vi "Ethernet Packet Generator for Testing.vi"() -> ()   [LabVIEW 2025]
uses:
  <vilib>/xnet/xnet.llb/XNET Frame Type Ethernet.ctl
  <vilib>/xnet/xnet.llb/XNET Create Session (Frame Output Stream).vi
  <vilib>/xnet/xnet.llb/XNET Write (Frame Ethernet).vi
  Automotive Ethernet Bus Monitor/Automotive Ethernet Bus Monitor.lvclass
panel:
  out "error out":errorcluster
  in  "Ethertype 3":u16=3 format="%.0x"
  in  "payload 3":string="medium payload"
  in  "Ethertype 2":u16=2 format="%.0x"
  in  "payload 2":string="payload1"
  in  "payload 1":string="payload2 is so much longer than payload1"
  in  "Ethertype 1":u16=1 format="%.0x"
  in  "destination MAC address":cluster{u8, u8, u8, u8, u8, u8}={255, 255, 255, 255, 255, 255} {"?" format="%.0x"; "?" format="%.0x"; "?" format="%.0x"; "?" format="%.0x"; "?" format="%.0x"; "?" format="%.0x"}
  in  "Has VLAN Tag 2":bool=TRUE
  in  "VID 2":u16=2
  in  "priority":u8=3
  in  "Stop":bool
  out "Number of Frames Sent":i32
  in  "Interface":refnum<k21>="ENET1"
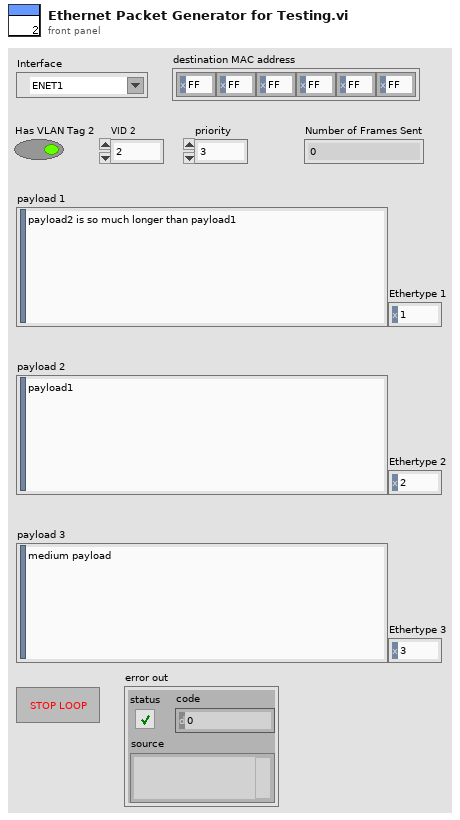
[diagram p1: front panel]
types:
  T1 = typedef "XNET Frame Type Ethernet.ctl" = u16
  T2 = cluster{"local timestamp":timestamp, "network timestamp":timestamp, "frame data":u8[], "fcs":u32, "type":T1, "network synced?":bool, "receive?":bool, "transmit?":bool, "error?":bool}
  T3 = cluster{"destination MAC address":cluster{u8, u8, u8, u8, u8, u8}, "source MAC address":cluster{u8, u8, u8, u8, u8, u8}, "Has VLAN Tag":bool, "VLAN Tag":cluster{"TPID":u16, "priority":u8, "DEI":bool, "VID":u16}, "Ethertype":u16}
  T4 = cluster{"TPID":u16, "priority":u8, "DEI":bool, "VID":u16}
  T5 = cluster{"local timestamp":timestamp, "network timestamp":timestamp, "frame data":u8[], "fcs":u32, "type":T1, "network synced?":bool, "receive?":bool, "transmit?":bool, "error?":bool}[]
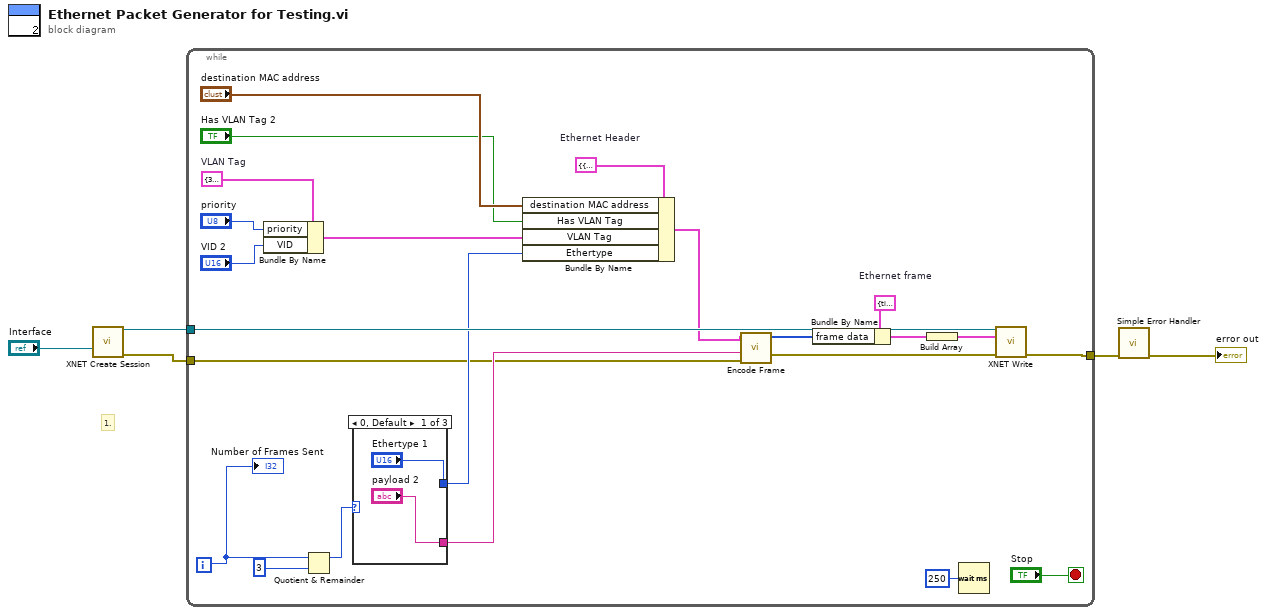
[diagram p0: block diagram]
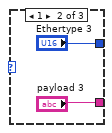
[diagram p2: hidden frame]
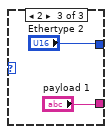
[diagram p3: hidden frame]
diagram:
  # "1."
  n1 = call-poly <vilib>:"XNET Create Session.vi"("interface"="Interface") -> ("session out"=w4:refnum<k21>, "error out"=w2:errorcluster)  [unwired: 13 in]
  n2 = while {
    tunnel: w4 -> [w28]
    tunnel: [w25] -> w3
    tunnel: w2 -> [w6]
    i -> [w12]
    stop <- "Stop" stop-if-true
    w19 = T2 {"local timestamp"=timestamp(0 s since 1904-01-01), "network timestamp"=timestamp(0 s since 1904-01-01), "frame data"=[], "fcs"=0, "type"=0, "network synced?"=FALSE, "receive?"=FALSE, "transmit?"=FALSE, "error?"=FALSE}  # Ethernet frame
    w24 = T3 {"destination MAC address"={0, 0, 0, 0, 0, 0}, "source MAC address"={0, 0, 0, 0, 0, 0}, "Has VLAN Tag"=FALSE, "VLAN Tag"={"TPID"=33024, "priority"=0, "DEI"=FALSE, "VID"=0}, "Ethertype"=0}  # Ethernet Header
    w23 = T4 {"TPID"=33024, "priority"=0, "DEI"=FALSE, "VID"=0}  # VLAN Tag
    n3 = Bundle By Name(cluster=w23, "priority"="priority", "VID"="VID 2") -> (w22:T4)
    n4 = Quotient & Remainder(x=w12, y=3) -> (x-y*floor(x/y)=w14:i32)  [unwired: 1 out]
    n5 = case shown="0, Default" w14 {
      tunnel: ["payload 2" "payload 3" "payload 1"] -> w8
      tunnel: ["Ethertype 1" "Ethertype 3" "Ethertype 2"] -> w11
      frame 0, Default {
      }
      frame 1 {
      }
      frame 2 {
      }
    }
    n6 = Bundle By Name(cluster=w24, "destination MAC address"="destination MAC address", "Has VLAN Tag"="Has VLAN Tag 2", "VLAN Tag"=w22, "Ethertype"=w11) -> (w10:T3)
    n7 = call "Encode Frame.vi"("error in (no error)"=w6, "payload"=w8, "Ethernet Header"=w10) -> ("error out"=w7:errorcluster, "frame data"=w9:u8[])  [unwired: 7 in]
    n8 = Bundle By Name(cluster=w19, "frame data"=w9) -> (w18:T2)
    n9 = Build Array(w18) -> (w17:T5)
    n10 = Wait (ms)(milliseconds to wait=u32 250) -> ()  [unwired: 1 out]
    n11 = call-poly <vilib>:"XNET Write.vi"("session in"=w28, "data"=w17, "error in (no error)"=w7) -> ("error out"=w25:errorcluster)  [unwired: 11 in, 1 out]
    "Number of Frames Sent" <- w12
  }
  n12 = call <vilib>:"Simple Error Handler.vi"("error in (no error)"=w3) -> ("error out"=→"error out":errorcluster)  [unwired: 4 in, 4 out]
